vi "Channel Selection Screen.vi"(7 "guids":string[](array[string])=["4b95dee7-8d64-48ce-932c-f5fdd14e4d4c", "94e87467-031b-484c-a85e-bcbac581524d"], 8 "error in":errorcluster, 10 "Selected Channels":T1, 11 "Parent Ref":T3=18446744073709551615 format="%.0x") -> (0 "error out":errorcluster, 1 "Cancelled?":bool, 2 "Selected Channels":T1, 3 "Parent Ref Out":T3=18446744073709551615 format="%.0x")   [LabVIEW 2019, in "Protection and Counter Support System Explorer.lvlib"]
uses:
  Protection and Counter Support System Explorer.lvlib
  NationalInstruments.VeriStand.SystemStorageUI
  <vilib>/NI VeriStand/Custom Device API/Custom Device Item Ref.ctl
  Types/Protection Signal Settings.ctl
  Types/Protection Signal Linked Channel.ctl
  Shared/Types/Protection Type.ctl
  <vilib>/NI VeriStand/Custom Device API/Custom Device API.lvlib
  Shared/Protection and Counter Support Shared.lvlib
panel:
  in  "Cancel":bool
  in  "OK":bool
  in  "Protection Data":refnum<k24>(container)
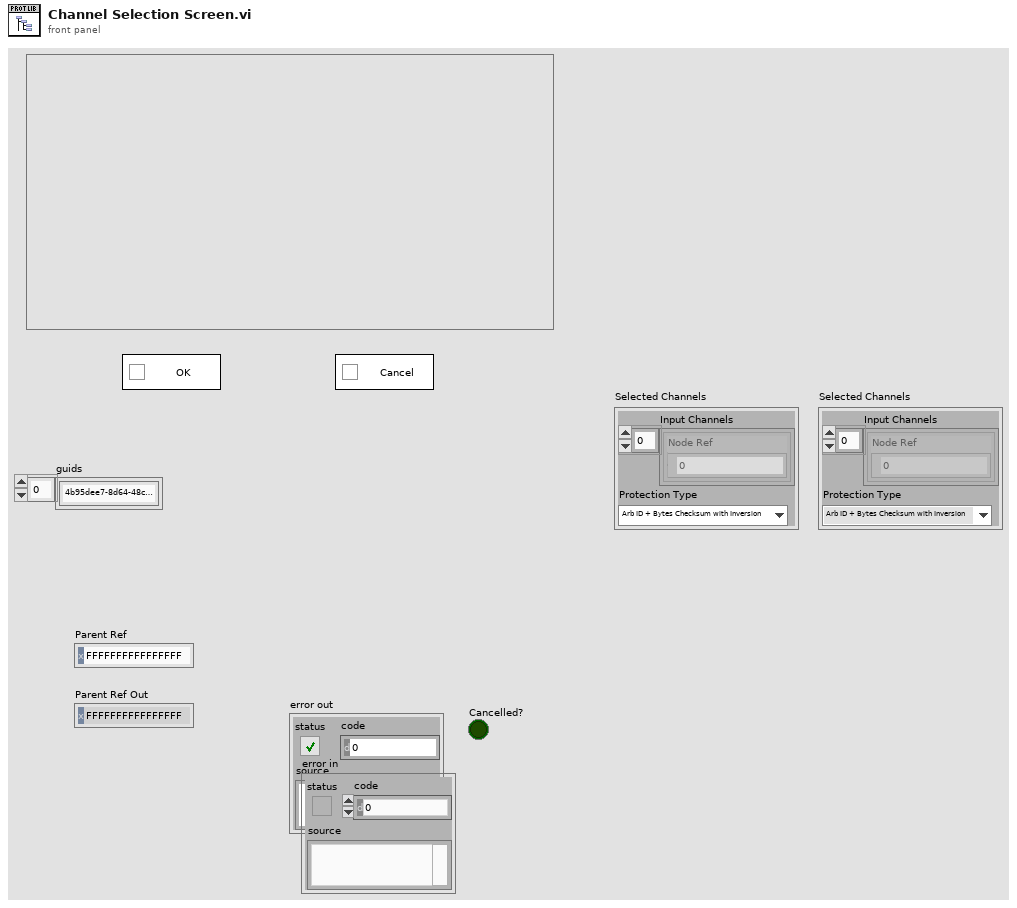
[diagram p1: front panel]
types:
  T1 = typedef "Protection and Counter Support System Explorer.lvlib/Protection Signal Settings.ctl" = cluster{"Input Channels":T2[], "Protection Type":T4}
  T2 = typedef "Protection and Counter Support System Explorer.lvlib/Protection Signal Linked Channel.ctl" = cluster{"Node Ref":T3}
  T3 = typedef "Custom Device API.lvlib/Custom Device Item Ref.ctl" = u64
  T4 = typedef "Protection and Counter Support Shared.lvlib/Protection Type.ctl" = enum16{"Arb ID + Bytes Checksum with Inversion", "Arb ID + Bytes CRC with Inversion", "Reversed Raw Signal Checksum with Inversion", "Concatenated Two's Compliment"}
  T5 = typedef "Custom Device API.lvlib/Custom Device Pointer.ctl" = refnum<k24>
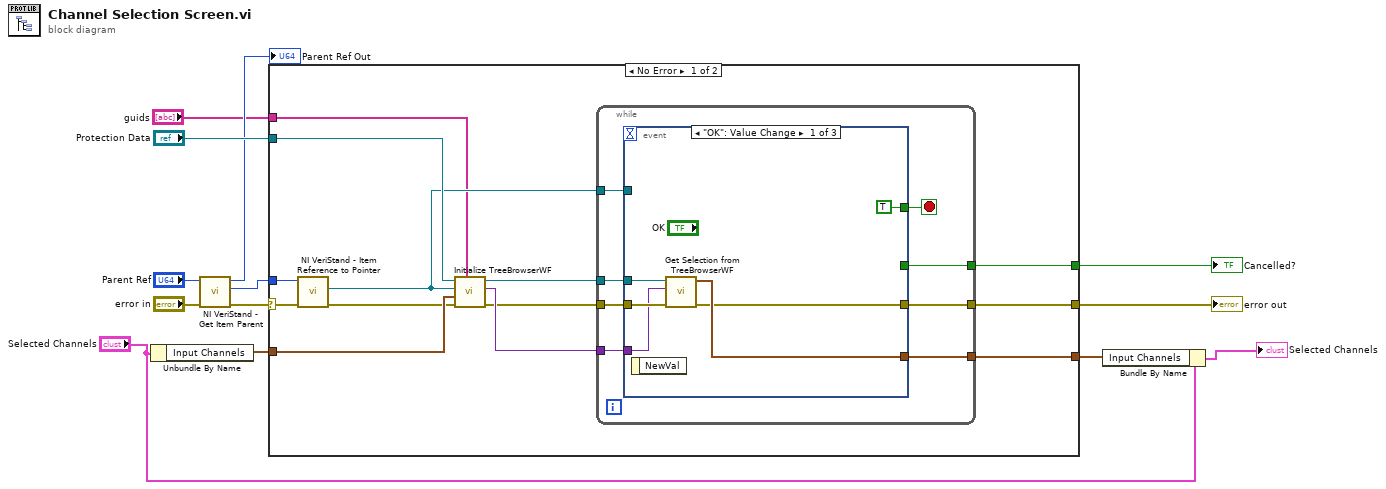
[diagram p0: block diagram]
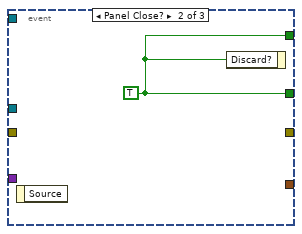
[diagram p2: hidden frame]
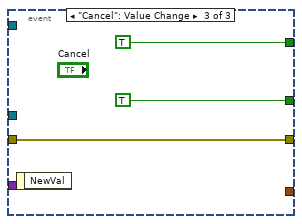
[diagram p3: hidden frame]
diagram:
  n1 = Unbundle By Name("Selected Channels") -> ("Input Channels"=w10:T2[])
  n2 = call <vilib>:"NI VeriStand - Get Item Parent.vi"("error in (no error)"="error in", "Item Ref in"="Parent Ref") -> ("error out"=w4:errorcluster, "Parent Ref"=w2:T3, "Item Ref out"=→"Parent Ref Out":T3)  [unwired: 6 in, 1 out]
  n3 = case shown="No Error" w4 {
    selector: w4 -> [w25 w45]
    tunnel: "Protection Data" -> [w21 _]
    tunnel: w2 -> [w26 _]
    tunnel: [w24 _] -> w12
    tunnel: [w18 w45] -> w11
    tunnel: [w23 _] -> w9
    tunnel: w10 -> [w22 _]
    tunnel: "guids" -> [w14 _]
    frame No Error {
      n4 = call <vilib>:"NI VeriStand - Item Reference to Pointer.vi"("error in (no error)"=w25, "Item Ref in"=w26) -> ("error out"=w17:errorcluster, "Node Pointer"=w16:T5)  [unwired: 6 in, 2 out]
      n5 = call "Initialize TreeBrowserWF.vi"("guids"=w14, "error in (no error)"=w17, "Input Channels"=w22, "Node Pointer"=w16, "TreeBrowserRef"=w21) -> ("error out"=w15:errorcluster, "Channels"=w20:variant, "TreeBrowserRef 2"=w19:refnum<k24>)  [unwired: 4 in]
      n6 = while {
        tunnel: w15 -> [w34]
        tunnel: w19 -> [w33]
        tunnel: [w31] -> w24
        tunnel: [w30] -> w18
        tunnel: [w29] -> w23
        tunnel: w20 -> [w28]
        tunnel: w16 -> [w27]
        stop <- w32 stop-if-true
        n7 = event shown="[0] \"OK\": Value Change" {
          selector: _ -> [_ _ _]
          dyn-events: _ -> [_ _ _]
          timeout: _ -> [_ _ _]
          tunnel: w34 -> [w40 _ w44]
          tunnel: w33 -> [w39 _ _]
          tunnel: [w36 _ w44] -> w30
          tunnel: [TRUE w41 TRUE] -> w32
          tunnel: [_ w41 TRUE] -> w31
          tunnel: [w37 _ _] -> w29
          tunnel: w28 -> [w38 _ _]
          tunnel: w27 -> [_ _ _]
          event "OK": Value Change {
            n8 = event-data() -> ()  [unwired: 1 in, 1 out]
            n9 = call "Get Selection from TreeBrowserWF.vi"("error in (no error)"=w40, "Input Channels"=w38, ".NET Refnum in"=w39) -> ("error out"=w36:errorcluster, "Input Channel Selections"=w37:T2[])  [unwired: 7 in]
          }
          event Panel Close? {
            w41 = TRUE
            n10 = event-data() -> ()  [unwired: 1 in, 1 out]
            n11 = event-data("Discard?"=w41) -> ()  [unwired: 1 in, 1 out]
          }
          event "Cancel": Value Change {
            n12 = event-data() -> ()  [unwired: 1 in, 1 out]
          }
        }
      }
    }
    frame Error {
    }
  }
  "Cancelled?" <- w12
  "error out" <- w11
  n13 = Bundle By Name(cluster="Selected Channels", "Input Channels"=w9) -> (→"Selected Channels":T1)
